vi "Record Frame.vi"(7 "Size per frame (bytes)":dbl, 8 "error in (no error)":errorcluster, 9 "Append":bool, 10 "Probe Position":T1, 11 "Frame Grabber Data In in":T5={"Camera Session"="", "Frame"=refnum, "AVI Refnum"=refnum, "Codecs"=[], "Frame number"=0, "Tracking File Refnum"=refnum, "Tick Count"=0, "Probe Object"=refnum, "Playback Probe Data"=[], "Rigid Body"={"Position"={"x (mm)"=0.0, "y (mm)"=0.0, "z (mm)"=0.0}, "Orientation"={"Pitch (rad)"=0.0, "Yaw (rad)"=0.0, "Roll (rad)"=0.0}, "Quaternion"={"qx"=0.0, "qy"=0.0, "qz"=0.0, "qw"=0.0}, "Tracked?"=FALSE}, "Total no frames playback"=0, "Video FPS"=0.0, "Camera connected?"=FALSE, "Scene"=refnum, "Cropped Frame"=refnum, "Tracker FPS"=0.0, "Crop ROI"=[], "Presentation Values"=[], "Elapsed time (ms)"=0, "Camera frames playback"=0, "Refnums"={"Live Refnum"=refnum, "Record Refnum"=refnum, "Recording Settings Refnum"=refnum, "Playback Refnum"=refnum, "Frame Slider Refnum"=refnum, "Pause Refnum"=refnum, "Home Refnum"=refnum, "Crop Refnum"=refnum, "Clear Crop Refnum"=refnum, "stop refnum"=refnum, "Playback Rate Refnum"=refnum, "Operator Settings Refnums"=refnum, "Presentation Refnum"=refnum, "Gestation Refnum"=refnum, "Connection Settings Refnum"=refnum, "Crop Time Frame Slider Refnum"=refnum}, "Dimensions"={"Probe Dimensions"={"Probe Width"=0.0, "Probe Depth"=1.0, "Probe Height"=0.0}, "Room Dimensions"={"Room Width"=0.0, "Room Depth"=0.0, "Room Height"=0.0}}, "Playback Data As Strings"=[], "Cropped Tracking File Refnum"=refnum, "Cropped AVI Refnum"=refnum}) -> (0 "error out":errorcluster, 1 "Time elapsed (s)":dbl, 2 "Image":T4, 3 "Frame Grabber Data out":T5={"Camera Session"="", "Frame"=refnum, "AVI Refnum"=refnum, "Codecs"=[], "Frame number"=0, "Tracking File Refnum"=refnum, "Tick Count"=0, "Probe Object"=refnum, "Playback Probe Data"=[], "Rigid Body"={"Position"={"x (mm)"=0.0, "y (mm)"=0.0, "z (mm)"=0.0}, "Orientation"={"Pitch (rad)"=0.0, "Yaw (rad)"=0.0, "Roll (rad)"=0.0}, "Quaternion"={"qx"=0.0, "qy"=0.0, "qz"=0.0, "qw"=0.0}, "Tracked?"=FALSE}, "Total no frames playback"=0, "Video FPS"=0.0, "Camera connected?"=FALSE, "Scene"=refnum, "Cropped Frame"=refnum, "Tracker FPS"=0.0, "Crop ROI"=[], "Presentation Values"=[], "Elapsed time (ms)"=0, "Camera frames playback"=0, "Refnums"={"Live Refnum"=refnum, "Record Refnum"=refnum, "Recording Settings Refnum"=refnum, "Playback Refnum"=refnum, "Frame Slider Refnum"=refnum, "Pause Refnum"=refnum, "Home Refnum"=refnum, "Crop Refnum"=refnum, "Clear Crop Refnum"=refnum, "stop refnum"=refnum, "Playback Rate Refnum"=refnum, "Operator Settings Refnums"=refnum, "Presentation Refnum"=refnum, "Gestation Refnum"=refnum, "Connection Settings Refnum"=refnum, "Crop Time Frame Slider Refnum"=refnum}, "Dimensions"={"Probe Dimensions"={"Probe Width"=0.0, "Probe Depth"=1.0, "Probe Height"=0.0}, "Room Dimensions"={"Room Width"=0.0, "Room Depth"=0.0, "Room Height"=0.0}}, "Playback Data As Strings"=[], "Cropped Tracking File Refnum"=refnum, "Cropped AVI Refnum"=refnum}, 5 "Greater than 2 GB?":bool)   [LabVIEW 2017]
uses:
  Controls/Frame Grabber Data.ctl
  <vilib>/userdefined/High Color/IMAQdx.ctl
  <vilib>/vision/Image Controls.llb/IMAQ Image.ctl
  <vilib>/vision/Avi.llb/IMAQ AVI2 Refnum.ctl
  Controls/Rigid Body Info.ctl
  Controls/Position.ctl
  Controls/Orientation.ctl
  Controls/Refnums.ctl
  Controls/Recording Settings.ctl
  Controls/Operator Settings.ctl
  Controls/Operator.ctl
  Controls/Dimensions.ctl
  Controls/Room Dimensions.ctl
panel:
  out "Camera frame number":dbl
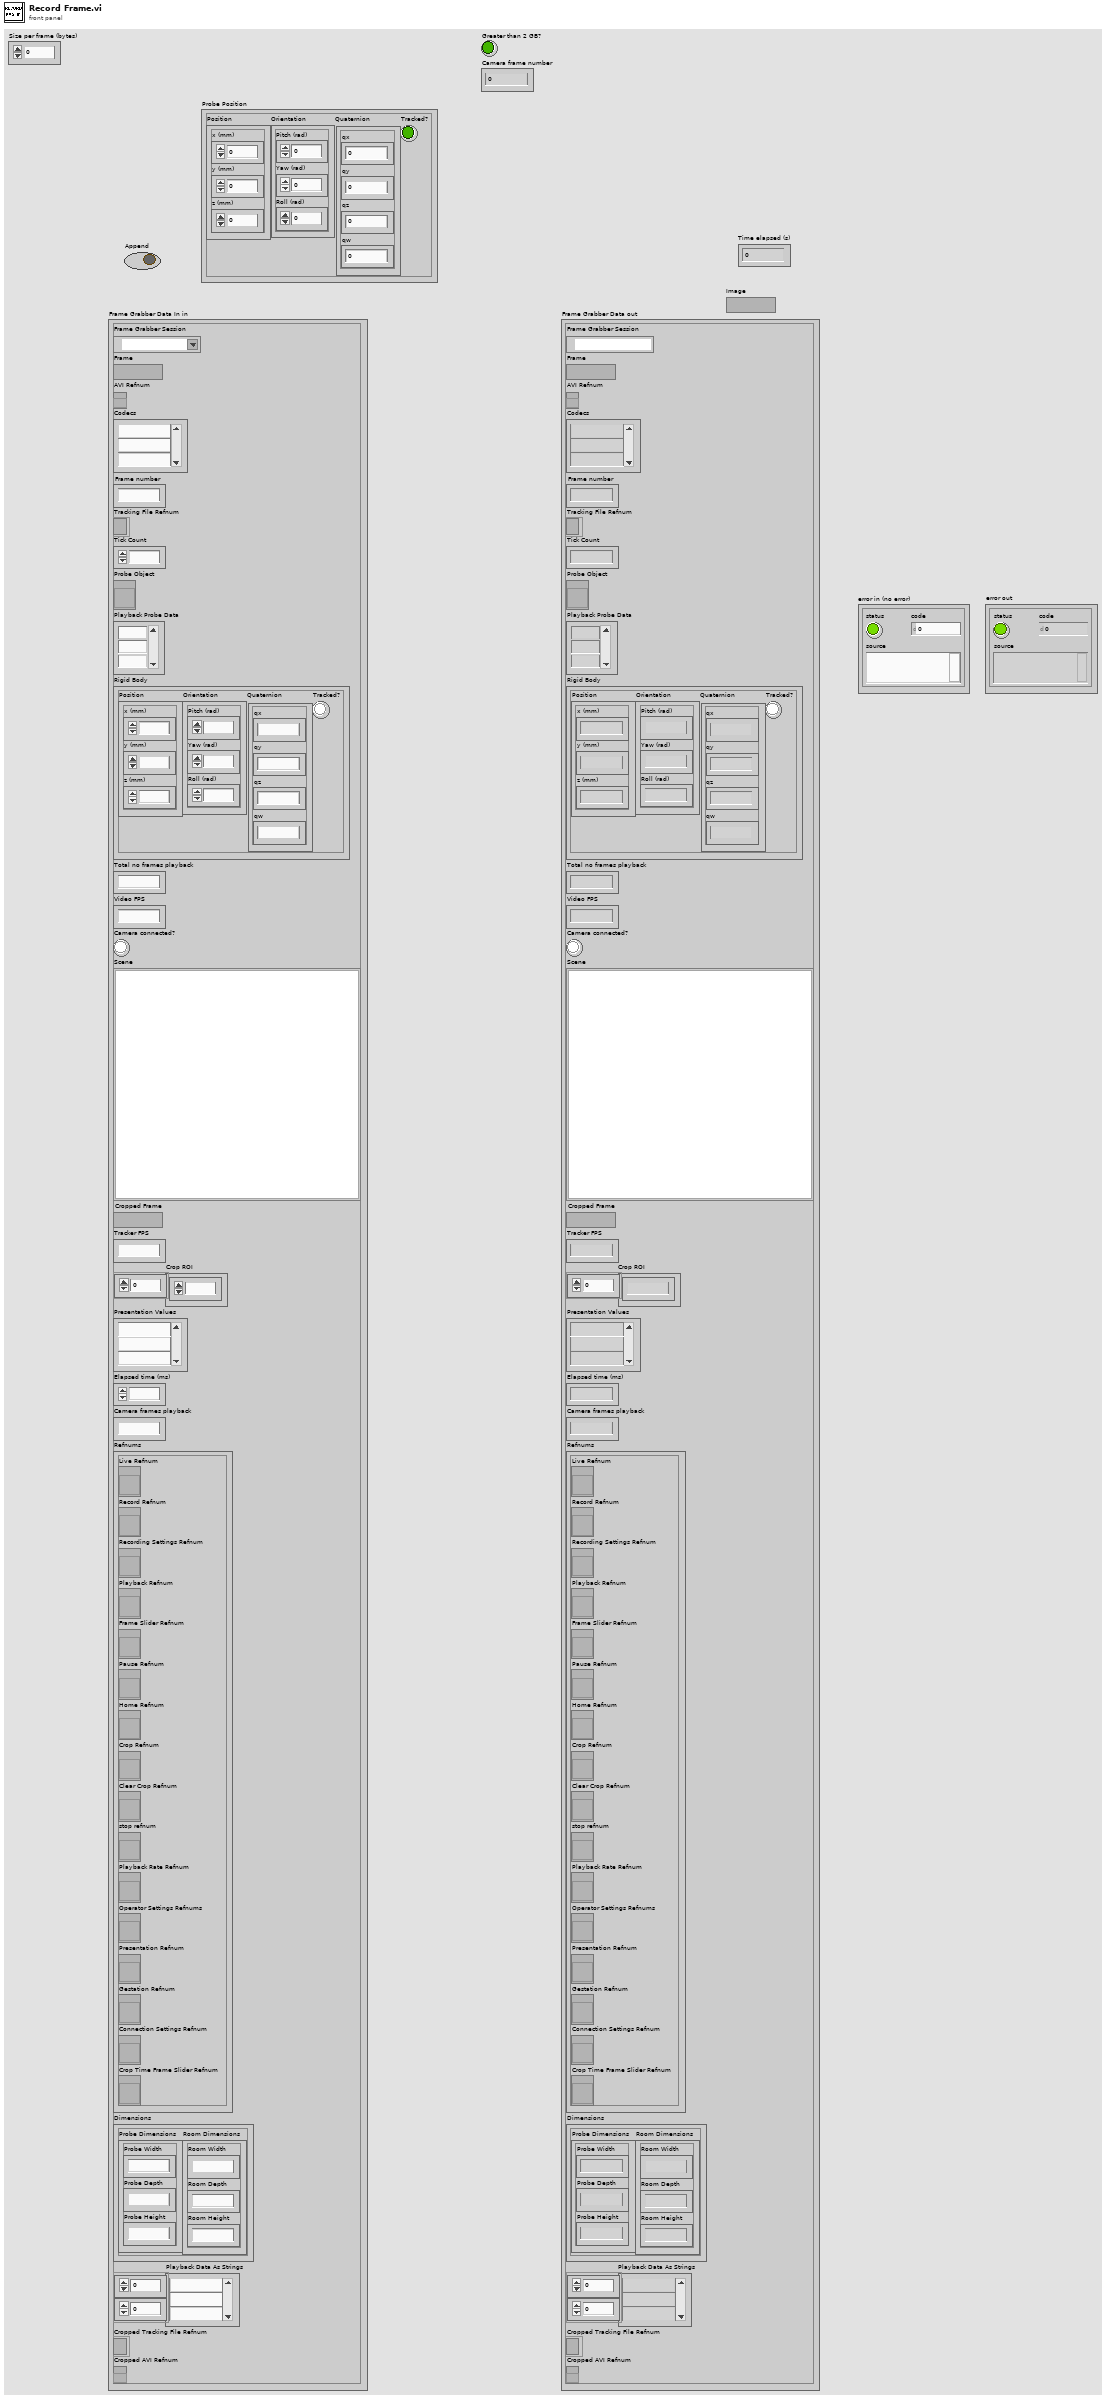
[diagram p1: front panel]
types:
  T1 = typedef "Rigid Body Info.ctl" = cluster{"Position":T2, "Orientation":T3, "Quaternion":cluster{"qx":sgl, "qy":sgl, "qz":sgl, "qw":sgl}, "Tracked?":bool}
  T2 = typedef "Position.ctl" = cluster{"x (mm)":sgl, "y (mm)":sgl, "z (mm)":sgl}
  T3 = typedef "Orientation.ctl" = cluster{"Pitch (rad)":sgl, "Yaw (rad)":sgl, "Roll (rad)":sgl}
  T4 = typedef "IMAQ Image.ctl" = refnum<image>
  T5 = typedef "Frame Grabber Data.ctl" = cluster{"Camera Session":T6, "Frame":T4, "AVI Refnum":T7, "Codecs":string[], "Frame number":u32, "Tracking File Refnum":refnum<file>, "Tick Count":u32, "Probe Object":refnum<vi>, "Playback Probe Data":dbl[][], "Rigid Body":T1, "Total no frames playback":i32, "Video FPS":dbl, "Camera connected?":bool, "Scene":refnum<vi>, "Cropped Frame":T4, "Tracker FPS":dbl, "Crop ROI":i32[], "Presentation Values":string[], "Elapsed time (ms)":u32, "Camera frames playback":u32, "Refnums":T8, "Dimensions":T9, "Playback Data As Strings":string[][], "Cropped Tracking File Refnum":refnum<file>, "Cropped AVI Refnum":T7}
  T6 = typedef "IMAQdx.ctl" = refnum<k21>
  T7 = typedef "IMAQ AVI2 Refnum.ctl" = refnum<k20>
  T8 = typedef "Refnums.ctl" = cluster{"Live Refnum":refnum<vi>, "Record Refnum":refnum<vi>, "Recording Settings Refnum":refnum<vi>, "Playback Refnum":refnum<vi>, "Frame Slider Refnum":refnum<vi>, "Pause Refnum":refnum<vi>, "Home Refnum":refnum<vi>, "Crop Refnum":refnum<vi>, "Clear Crop Refnum":refnum<vi>, "stop refnum":refnum<vi>, "Playback Rate Refnum":refnum<vi>, "Operator Settings Refnums":refnum<vi>, "Presentation Refnum":refnum<vi>, "Gestation Refnum":refnum<vi>, "Connection Settings Refnum":refnum<vi>, "Crop Time Frame Slider Refnum":refnum<vi>}
  T9 = typedef "Dimensions.ctl" = cluster{"Probe Dimensions":cluster{"Probe Width":sgl, "Probe Depth":sgl, "Probe Height":sgl}, "Room Dimensions":T10}
  T10 = typedef "Room Dimensions.ctl" = cluster{"Room Width":dbl, "Room Depth":dbl, "Room Height":dbl}
  T11 = typedef "Recording Settings.ctl" = cluster{"Folder to Save Recording":path, "Recording Name":string, "Video FPS":dbl, "Codec":u16, "Tracker FPS":dbl}
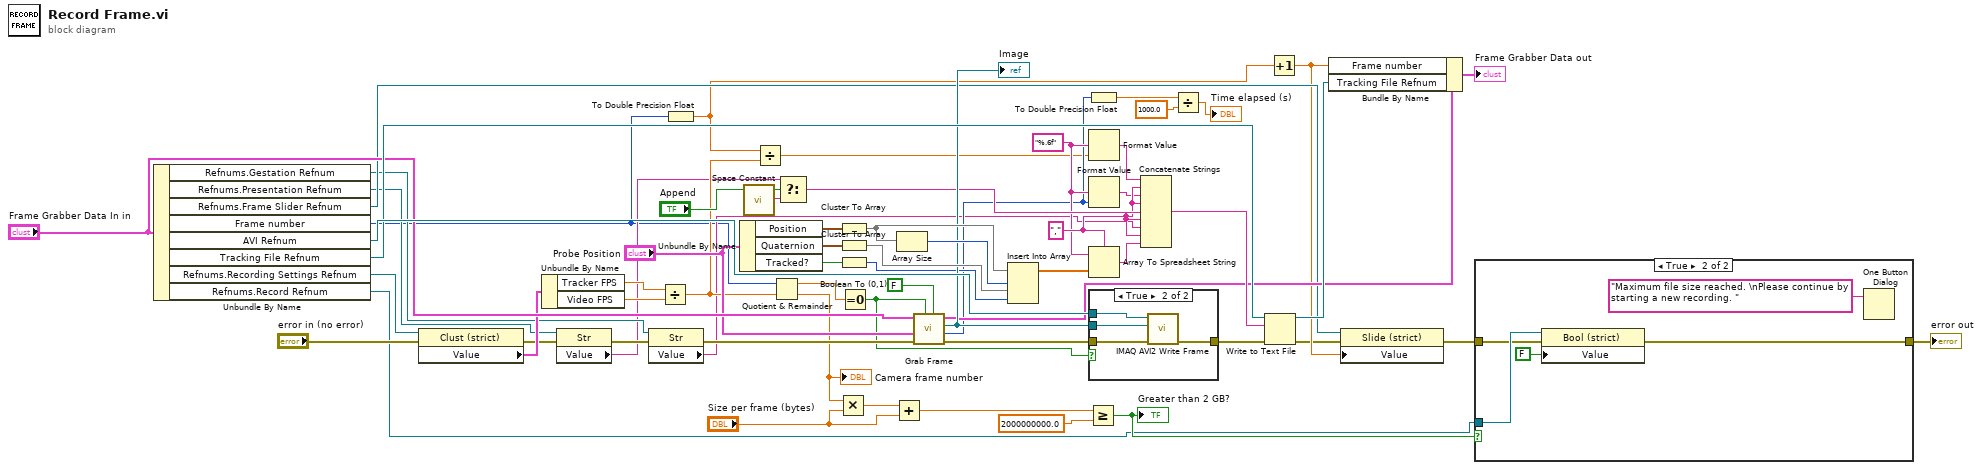
[diagram p0: block diagram]
diagram:
  w30 = "," ("delimiter (Tab)")
  w29 = "%.6f" ("format string")
  n1 = Unbundle By Name("Frame Grabber Data In in") -> ("Refnums.Gestation Refnum"=w19:refnum<vi>, "Refnums.Presentation Refnum"=w20:refnum<vi>, "Refnums.Frame Slider Refnum"=w42:refnum<vi>, "Frame number"=w11:u32, "AVI Refnum"=w61:T7, "Tracking File Refnum"=w60:refnum<file>, "Refnums.Recording Settings Refnum"=w23:refnum<vi>, "Refnums.Record Refnum"=w1:refnum<vi>)
  n2 = property class="Clust (strict)"(reference=w23, error in="error in (no error)") -> (error out=w18:errorcluster, "Value"=w22:T11)  [unwired: 1 out]
  n3 = Unbundle By Name(w22) -> ("Tracker FPS"=w38:dbl, "Video FPS"=w35:dbl)
  n4 = property class="Str"(reference=w20, error in=w18) -> (error out=w17:errorcluster, "Value"=w14:string)  [unwired: 1 out]
  n5 = property class="Str"(reference=w19, error in=w17) -> (error out=w16:errorcluster, "Value"=w15:string)  [unwired: 1 out]
  n6 = Divide(x=w38, y=w35) -> (x/y=w31:dbl)
  n7 = To Double Precision Float(number=w11) -> (double precision float=w13:dbl)
  n8 = Unbundle By Name("Probe Position") -> ("Position"=w54:T2, "Quaternion"=w58:cluster{"qx":sgl, "qy":sgl, "qz":sgl, "qw":sgl}, "Tracked?"=w44:bool)
  n9 = call <vilib>:"Space Constant.vi"() -> ("String"=w39:string)
  n10 = Divide(x=w13, y=w31) -> (x/y=w12:dbl)
  n11 = Quotient & Remainder(x=w11, y=w31) -> (x-y*floor(x/y)=w36:dbl, floor(x/y)=w9:dbl)
  "Camera frame number" <- w9
  n12 = Select(t=w14, s="Append", f=w39) -> (s? t:f=w32:string)
  n13 = Multiply(x=w9, y="Size per frame (bytes)") -> (x*y=w8:dbl)
  n14 = Cluster To Array(cluster=w54) -> (array=w56:sgl[])
  n15 = Cluster To Array(cluster=w58) -> (array=w55:sgl[])
  n16 = Boolean To (0,1)(Boolean=w44) -> (0, 1=w43:i16)
  n17 = Equal To 0?(x=w36) -> (x = 0?=w10:bool)
  n18 = Add(x=w8, y="Size per frame (bytes)") -> (x+y=w6:dbl)
  n19 = Array Size(array=w56) -> (size(s)=w57:i32)
  n20 = call "Grab Frame.vi"("Live?"=FALSE, "Grab frame?"=w10, "error in (no error)"=w16, "Rigid Body"="Probe Position", "Frame Grabber Data in"="Frame Grabber Data In in") -> ("error out"=w49:errorcluster, "Elapsed time (ms)"=w27:u32, "Frame"=w50:T4, "Frame Grabber Data out"=w46:T5)  [unwired: 3 in]
  "Image" <- w50
  n21 = Insert Into Array(array=w56, index=w57, new element #1=w55, new element #2=w43) -> (w59:sgl[])
  n22 = Greater Or Equal?(x=w6, y=2000000000.0) -> (x >= y?=w4:bool)
  "Greater than 2 GB?" <- w4
  n23 = To Double Precision Float(number=w27) -> (double precision float=w25:dbl)
  n24 = Format Value(format string=w29, value (0)=w12) -> (output string=w33:string)  [unwired: 1 in]
  n25 = Format Value(format string=w29, value (0)=w27) -> (output string=w28:string)  [unwired: 1 in]
  n26 = Array To Spreadsheet String(delimiter (Tab)=w30, array=w59, 3:w29) -> (spreadsheet string=w53:string)
  n27 = case shown="True" w10 {
    tunnel: [w63 w67] -> w62
    tunnel: w61 -> [_ w66]
    tunnel: w50 -> [_ w65]
    tunnel: w49 -> [w63 w64]
    frame False {
    }
    frame True {
      n28 = call "IMAQ AVI2 Write Frame"("error in (no error)"=w64, "Image"=w65, "AVI Refnum"=w66) -> ("error out"=w67:errorcluster)  [unwired: 6 in, 2 out]
    }
  }
  n29 = Concatenate Strings(w33, w30, w28, w30, w32, w30, w15, w30, w53) -> (w52:string)
  n30 = Divide(x=w25, y=1000.0) -> (x/y=→"Time elapsed (s)":dbl)
  n31 = Write to Text File(file (use dialog)=w60, text=w52, error in=w62) -> (refnum out=w51:refnum<file>, error out=w40:errorcluster)  [unwired: 1 in, 1 out]
  n32 = Increment(x=w13) -> (x+1=w41:dbl)
  n33 = Bundle By Name(cluster=w46, "Frame number"=w41, "Tracking File Refnum"=w51) -> (→"Frame Grabber Data out":T5)
  n34 = property class="Slide (strict)"(reference=w42, error in=w40, "Value"=w41) -> (error out=w3:errorcluster)  [unwired: 1 out]
  n35 = case shown="True" w4 {
    tunnel: w3 -> [w68 w71]
    tunnel: [w68 w70] -> w2
    tunnel: w1 -> [_ w72]
    frame False {
    }
    frame True {
      n36 = property class="Bool (strict)"(reference=w72, error in=w71, "Value"=FALSE) -> (error out=w70:errorcluster)  [unwired: 1 out]
      n37 = One Button Dialog(message="Maximum file size reached. \nPlease continue by starting a new recording. ") -> ()  [unwired: 1 in, 1 out]
    }
  }
  "error out" <- w2
